vi "Main_DataFGVTest.vi"() -> ()   [LabVIEW 2015]
uses:
  control_DataFGVTest.ctl
  <userlib>/FGV/control/Control_Data.ctl
panel:
  out "element":T1
  in  "Action":T2
  in  "data":i32
  in  "file (use dialog)":path=path "D:/dataFGV"
  out "error out":errorcluster
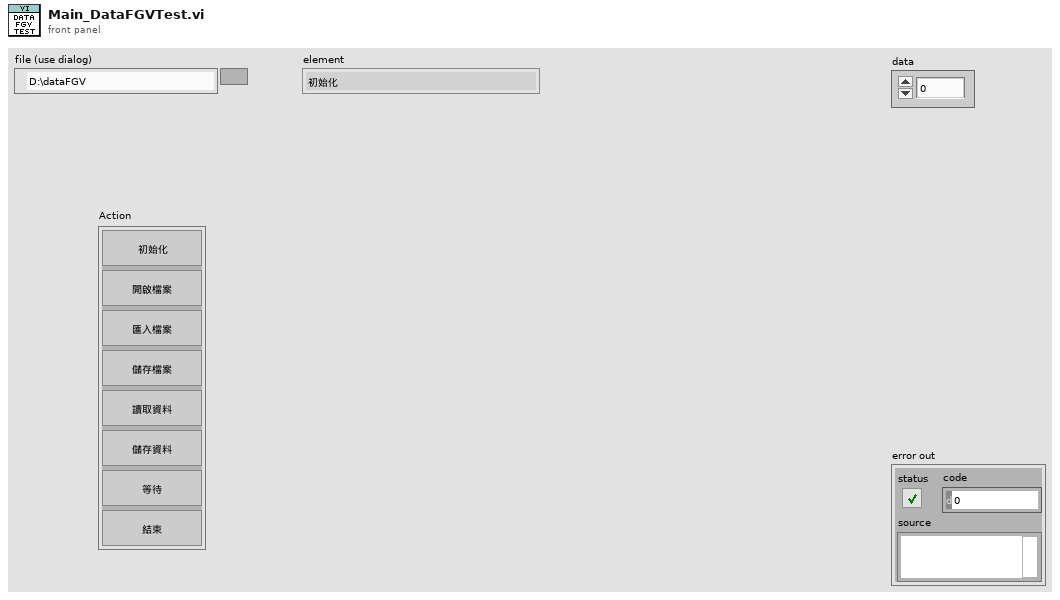
[diagram p1: front panel]
types:
  T1 = typedef "control_DataFGVTest.ctl" = enum16{"初始化", "開啟檔案", "匯入檔案", "儲存檔案", "讀取資料", "儲存資料", "等待", "結束"}
  T2 = cluster{"初始化":bool, "開啟檔案":bool, "匯入檔案":bool, "儲存檔案":bool, "讀取資料":bool, "儲存資料":bool, "等待":bool, "結束":bool}
  T3 = typedef "Control_Data.ctl" = enum16{"Initialize", "Get Data", "Set Data", "Delete Data", "Idle"}
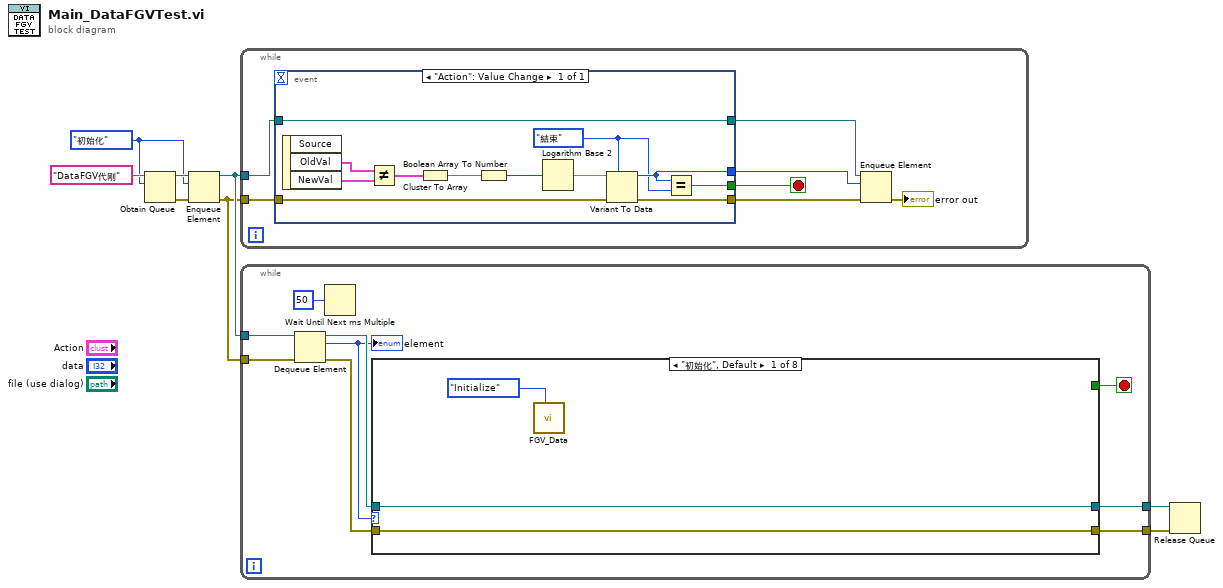
[diagram p0: block diagram]
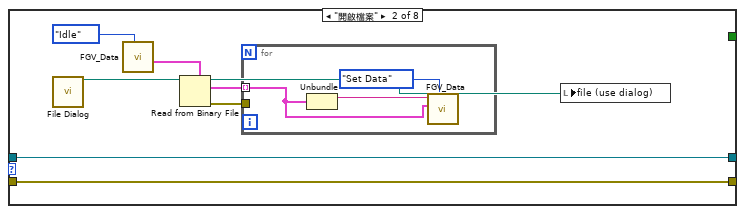
[diagram p2: hidden frame]
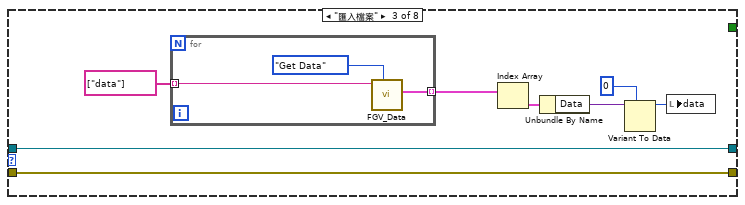
[diagram p3: hidden frame]
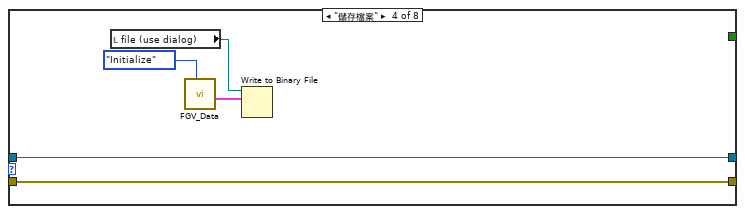
[diagram p4: hidden frame]
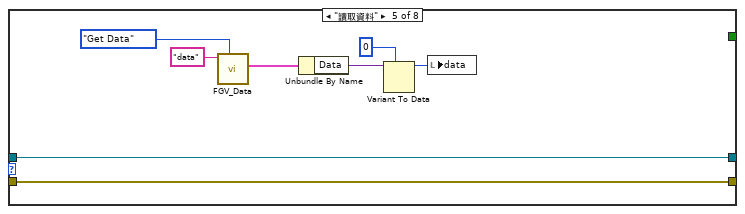
[diagram p5: hidden frame]
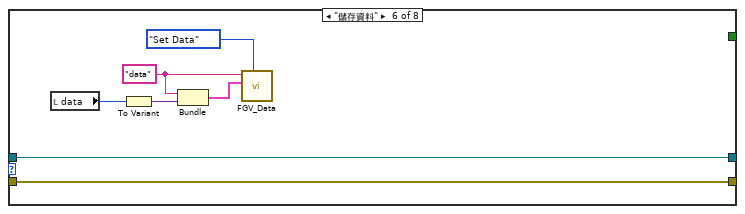
[diagram p6: hidden frame]
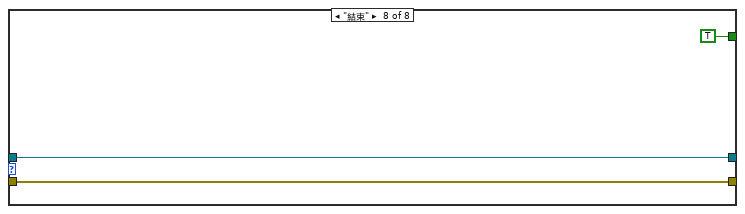
[diagram p8: hidden frame]
diagram:
  w1 = control_DataFGVTest."初始化" ("Enum")
  n1 = Obtain Queue(name (unnamed)="DataFGV代刚", element data type=w1) -> (queue out=w7:refnum<queue>, error out=w6:errorcluster)  [unwired: 3 in, 1 out]
  n2 = Enqueue Element(queue=w7, element=w1, error in (no error)=w6) -> (queue out=w3:refnum<queue>, error out=w2:errorcluster)  [unwired: 1 in, 1 out]
  n3 = while {
    tunnel: w2 -> [w15]
    tunnel: w3 -> [w14]
    stop <- w11 stop-if-true
    n4 = event shown="[0] \"Action\": Value Change" {
      selector: _ -> [_]
      dyn-events: _ -> [_]
      timeout: _ -> [_]
      tunnel: w15 -> [w17]
      tunnel: w14 -> [w21]
      tunnel: [w18] -> w13
      tunnel: [w21] -> w12
      tunnel: [w19] -> w11
      tunnel: [w20] -> w9
      event "Action": Value Change {
        w16 = control_DataFGVTest."結束" ("Enum")
        n5 = event-data() -> ("OldVal"=w27:T2, "NewVal"=w26:T2)  [unwired: 1 in, 1 out]
        n6 = Not Equal?(x=w27, y=w26) -> (x != y?=w25:T2)
        n7 = Cluster To Array(cluster=w25) -> (array=w24:bool[])
        n8 = Boolean Array To Number(Boolean array=w24) -> (number=w23:u32)
        n9 = Logarithm Base 2(1:w23) -> (0:w22:dbl)
        n10 = Variant To Data(error in=w17, type=w16, Variant=w22) -> (data=w20:T1, error out=w18:errorcluster)
        n11 = Equal?(x=w20, y=w16) -> (x = y?=w19:bool)
      }
    }
    n12 = Enqueue Element(queue=w12, element=w9, error in (no error)=w13) -> (error out=→"error out":errorcluster)  [unwired: 1 in, 2 out]
  }
  n13 = while {
    tunnel: [w35] -> w5
    tunnel: w2 -> [w33]
    tunnel: w3 -> [w32]
    tunnel: [w31] -> w4
    stop <- w29 stop-if-true
    n14 = Dequeue Element(queue=w32, error in (no error)=w33) -> (queue out=w36:refnum<queue>, element=w28:T1, error out=w34:errorcluster)  [unwired: 1 in, 1 out]
    "element" <- w28
    n15 = Wait Until Next ms Multiple(millisecond multiple=u32 50) -> ()  [unwired: 1 out]
    n16 = case shown="\"初始化\", Default" w28 {
      tunnel: [w39 w46 w57 w65 w73 w80 w82 w85] -> w35
      tunnel: w36 -> [w39 w46 w57 w65 w73 w80 w82 w85]
      tunnel: w34 -> [w38 w45 w56 w64 w72 w79 w81 w84]
      tunnel: [w38 w45 w56 w64 w72 w79 w81 w84] -> w31
      tunnel: [_ _ _ _ _ _ _ TRUE] -> w29
      frame "初始化", Default {
        n17 = call <userlib>:"FGV_Data.vi"("Action_Data"=Control_Data."Initialize") -> ()  [unwired: 8 in, 3 out]
      }
      frame "開啟檔案" {
        n18 = call "File Dialog"() -> ("selected path"=w40:path)  [unwired: 12 in, 3 out]
        n19 = call <userlib>:"FGV_Data.vi"("Action_Data"=Control_Data."Idle") -> ("Data Array out"=w42:cluster{"Data name":string, "Data":variant}[])  [unwired: 8 in, 2 out]
        n20 = Read from Binary File(5:w42, 11:w40) -> (0:w44:errorcluster, 2:w43:cluster{"Data name":string, "Data":variant}[])  [unwired: 4 in, 2 out]
        n21 = for {
          tunnel: w43 -> [w48] mode=indexing
          tunnel: w44 -> [_]
          n22 = Unbundle(w48) -> ("Data name"=w49:string)  [unwired: 1 out]
          n23 = call <userlib>:"FGV_Data.vi"("Action_Data"=Control_Data."Set Data", "Data In"=w48, "Data name"=w49) -> ()  [unwired: 6 in, 3 out]
        }
        n24 = local write "file (use dialog)"(w40) -> ()
      }
      frame "匯入檔案" {
        n25 = for {
          tunnel: string[] ["data"] -> [w59] mode=indexing
          tunnel: [w58] -> w50 mode=indexing
          n26 = call <userlib>:"FGV_Data.vi"("Action_Data"=Control_Data."Get Data", "Data name"=w59) -> ("Data  Out"=w58:cluster{"Data name":string, "Data":variant})  [unwired: 7 in, 2 out]
        }
        n27 = Index Array(array=w50) -> (element=w54:cluster{"Data name":string, "Data":variant})  [unwired: 1 in]
        n28 = Unbundle By Name(w54) -> ("Data"=w53:variant)
        n29 = Variant To Data(type=0, Variant=w53) -> (data=w51:i32)  [unwired: 1 in, 1 out]
        n30 = local write "data"(w51) -> ()
      }
      frame "儲存檔案" {
        n31 = local read "file (use dialog)"() -> (w63:path)
        n32 = call <userlib>:"FGV_Data.vi"("Action_Data"=Control_Data."Initialize") -> ("Data Array out"=w62:cluster{"Data name":string, "Data":variant}[])  [unwired: 8 in, 2 out]
        n33 = Write to Binary File(file (use dialog)=w63, data=w62) -> ()  [unwired: 4 in, 3 out]
      }
      frame "讀取資料" {
        n34 = call <userlib>:"FGV_Data.vi"("Action_Data"=Control_Data."Get Data", "Data name"="data") -> ("Data  Out"=w66:cluster{"Data name":string, "Data":variant})  [unwired: 7 in, 2 out]
        n35 = Unbundle By Name(w66) -> ("Data"=w69:variant)
        n36 = Variant To Data(type=0, Variant=w69) -> (data=w67:i32)  [unwired: 1 in, 1 out]
        n37 = local write "data"(w67) -> ()
      }
      frame "儲存資料" {
        w74 = "data" ("Data name")
        n38 = local read "data"() -> (w77:i32)
        n39 = To Variant(anything=w77) -> (Variant=w76:variant)
        n40 = Bundle("Data name"=w74, "Variant"=w76) -> (w75:cluster{"Data name":string, "Variant":variant})  [unwired: 1 in]
        n41 = call <userlib>:"FGV_Data.vi"("Action_Data"=Control_Data."Set Data", "Data In"=w75, "Data name"=w74) -> ()  [unwired: 6 in, 3 out]
      }
      frame "等待" {
      }
      frame "結束" {
      }
    }
  }
  n42 = Release Queue(queue=w5, error in (no error)=w4) -> ()  [unwired: 1 in, 3 out]
